vi "Append error - WRITE.vi"(8 "error in (no error)":errorcluster, 9 "error":errorcluster, 11 "Simulated_CCD_Camera in":refnum<class "Sim_Ixon_Ultra.lvclass">) -> (0 "error out":errorcluster, 3 "Simulated_CCD_Camera out":refnum<class "Sim_Ixon_Ultra.lvclass">)   [LabVIEW 2018]
doc: "Append an error to the array of errors of the class\n\nThis array is verified before the start of an exposure. If an error is found, the exposure will not occur."
uses:
  Sim_Ixon_Ultra.lvclass
  C:/Users/Denis/Desktop/S4ACS/S4ACS/Simulated_CCD_Camera/Simulated Camera.lvclass
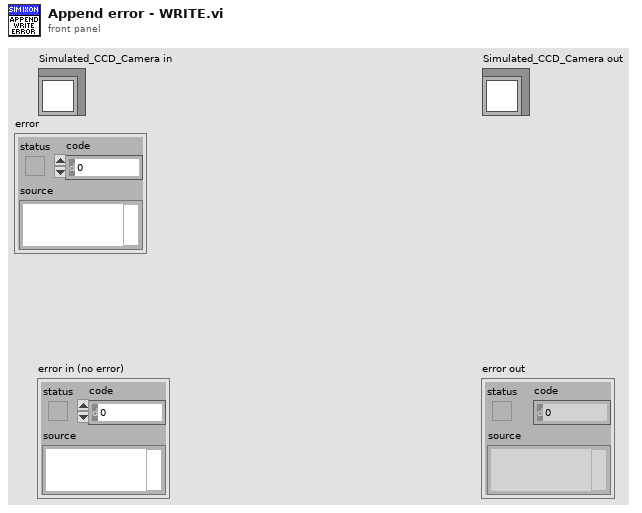
[diagram p1: front panel]
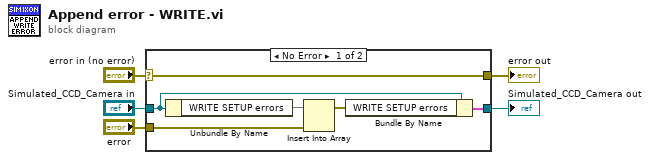
[diagram p0: block diagram]
diagram:
  n1 = case shown="No Error" "error in (no error)" {
    selector: "error in (no error)" -> [w11 w13]
    tunnel: [w11 w13] -> w4
    tunnel: [w9 w12] -> w2
    tunnel: "Simulated_CCD_Camera in" -> [w10 w12]
    tunnel: "error" -> [w8 _]
    frame No Error {
      n2 = Unbundle By Name(w10) -> ("WRITE SETUP errors"=w6)
      n3 = Insert Into Array(array=w6, new element=w8) -> (w7:errorcluster[])  [unwired: 1 in]
      n4 = Bundle By Name(cluster=w10, "WRITE SETUP errors"=w7) -> (w9:cluster{})
    }
    frame Error {
    }
  }
  "error out" <- w4
  "Simulated_CCD_Camera out" <- w2
